vi "Correct Deadtime.vi"(8 "error in (no error)":errorcluster, 9 "DT":dbl, 10 "LT":dbl, 11 "Raw Rate":dbl) -> (0 "error out":errorcluster, 2 "Corrected Rate":dbl)   [LabVIEW 2011]
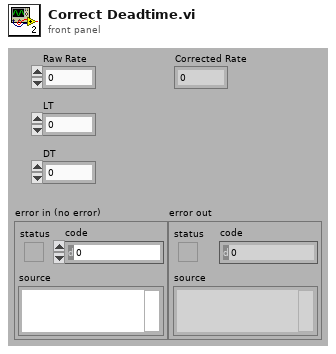
[diagram p1: front panel]
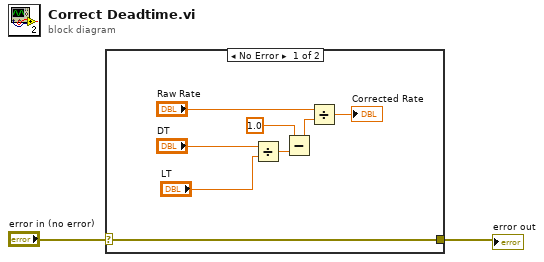
[diagram p0: block diagram]
diagram:
  n1 = case shown="No Error" "error in (no error)" {
    selector: "error in (no error)" -> [w3 w11]
    tunnel: [w3 w11] -> w1
    frame No Error {
      n2 = Divide(x="DT", y="LT") -> (x/y=w7:dbl)
      n3 = Subtract(x=1.0, y=w7) -> (x-y=w9:dbl)
      n4 = Divide(x="Raw Rate", y=w9) -> (x/y=→"Corrected Rate":dbl)
    }
    frame Error {
    }
  }
  "error out" <- w1
